vi "Data Acq Com.vi"(1 "command text in":string[](array[string]), 2 "option":T2) -> (0 "Command text out":string[][](array[string]))   [LabVIEW 2020]
uses:
  Ctl/option.ctl
  Data Acq.ctl
panel:
  in  "Data Acq":T1={"New/Stop File"=enum."New File", "Comments Option"=FALSE, "Comments"="", "extra wait"=5} {"extra wait" min=0}
  in  "cancel":bool
  in  "enter":bool
  # "Data Acquisition Program Control"
  # "AND wait extra"
  # "seconds"
  # "Advanced Control"
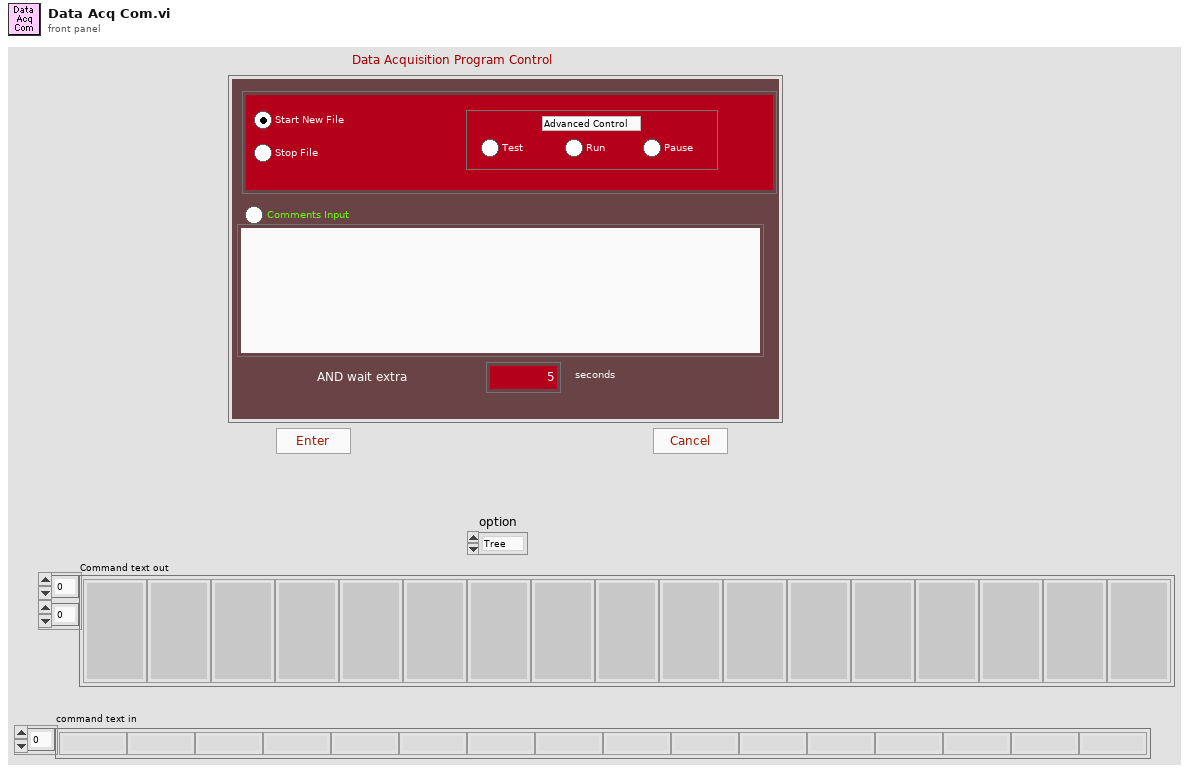
[diagram p1: front panel]
types:
  T1 = typedef "Data Acq.ctl" = cluster{"New/Stop File":enum32{"New File", "Stop FIle", "Test", "Run", "Pause"}, "Comments Option":bool, "Comments":string, "extra wait":i32}
  T2 = typedef "option.ctl" = enum16{"Tree", "List"}
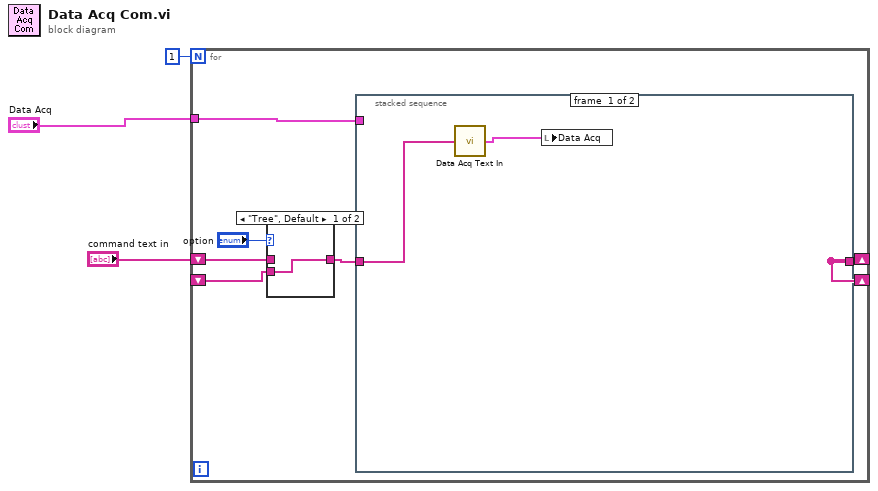
[diagram p0: block diagram]
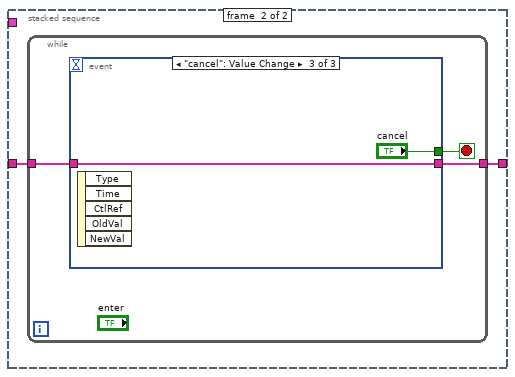
[diagram p3: hidden frame]
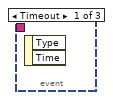
[diagram p4: hidden frame]
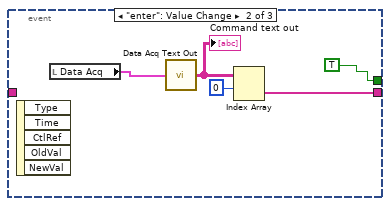
[diagram p5: hidden frame]
diagram:
  n1 = for {
    N: 1 -> [_]
    shift-right: [w4] -> _
    shift-left: _ -> [w8]
    shift-right: [w4] -> _
    shift-left: "command text in" -> [w7]
    tunnel: "Data Acq" -> [w5]
    n2 = case shown="\"Tree\", Default" "option" {
      tunnel: [w10 w11] -> w9
      tunnel: w8 -> [w10 _]
      tunnel: w7 -> [_ w11]
      frame "Tree", Default {
      }
      frame "List" {
      }
    }
    n3 = stacked-sequence {
      tunnel: [_ w15] -> w4
      tunnel: w9 -> [w12 w14]
      tunnel: w5 -> [_ _]
      frame #0 {
        n4 = call "Data Acq Text In.vi"("command text in"=w12) -> ("Data Acq"=w13:T1)
        n5 = local write "Data Acq"(w13) -> ()
      }
      frame #1 {
        n6 = while {
          tunnel: [w17] -> w15
          tunnel: w14 -> [w16]
          stop <- w18 stop-if-true
          n7 = event shown="[2] \"cancel\": Value Change" {
            selector: _ -> [_ _ _]
            dyn-events: _ -> [_ _ _]
            timeout: _ -> [_ _ _]
            tunnel: [_ TRUE "cancel"] -> w18
            tunnel: [_ w21 w24] -> w17
            tunnel: w16 -> [_ _ w24]
            event Timeout {
              n8 = event-data() -> ()  [unwired: 1 in, 2 out]
            }
            event "enter": Value Change {
              n9 = event-data() -> ()  [unwired: 1 in, 5 out]
              n10 = local read "Data Acq"() -> (w23:T1)
              n11 = call "Data Acq Text Out.vi"("Data Acq"=w23) -> ("Command text"=w22:string[][])
              "Command text out" <- w22
              n12 = Index Array(array=w22, index (row)=0 ("disabled index (col)")) -> (element=w21:string[])  [unwired: 1 in]
            }
            event "cancel": Value Change {
              n13 = event-data() -> ()  [unwired: 1 in, 5 out]
            }
          }
        }
      }
    }
  }
